vi "SamsGrapher.vi"() -> ()   [LabVIEW 2016]
uses:
  inventory type def.ctl
  Communication Global variables.vi
  <vilib>/addons/_JKI.lib/Serialization/JSON/JKI JSON Serialization.lvlib
panel:
  in  "Tab Control":enum32{"Controls", "Graph", "Help", "Fun"}(tab)
  in  "Load Config file":bool
  in  "Save Config file":bool
  in  "refresh list":bool
  in  "Device selection":i32(listbox)
  in  "Selected parameters":i32[](listbox)
  in  "Available parameters":i32[](listbox)
  in  "Config Button":bool
  out "Time range (Sec)":dbl format="%#.3g"
  in  "zoom out":bool
  in  "zoom in":bool
  out "Data rate (hz)":dbl(knob) scale=0.0..600.0
  in  "Enable graphing":bool=TRUE
  out "Waveform chart":waveform(dbl)[](graph)=[{"t0"=timestamp(742.987 s since 1904-01-01), "dt"=1.0, "Y"=[15300.0]}, {"t0"=timestamp(742.987 s since 1904-01-01), "dt"=1.0, "Y"=[15460.0]}, {"t0"=timestamp(742.987 s since 1904-01-01), "dt"=1.0, "Y"=[19658.0]}, {"t0"=timestamp(742.987 s since 1904-01-01), "dt"=1.0, "Y"=[18856.0]}]
  in  "stop":bool
  in  "Robor approved":u16(ring)
  in  "Robot Approved?":bool
  out "initialize error":errorcluster
  out "error out":errorcluster
  # "Parameter Selection"
  # "Xl Version 19.1.4"
  # "Click and drag \nselected parameters\nto change the order"
  # "Double click parameter name to add or remove it"
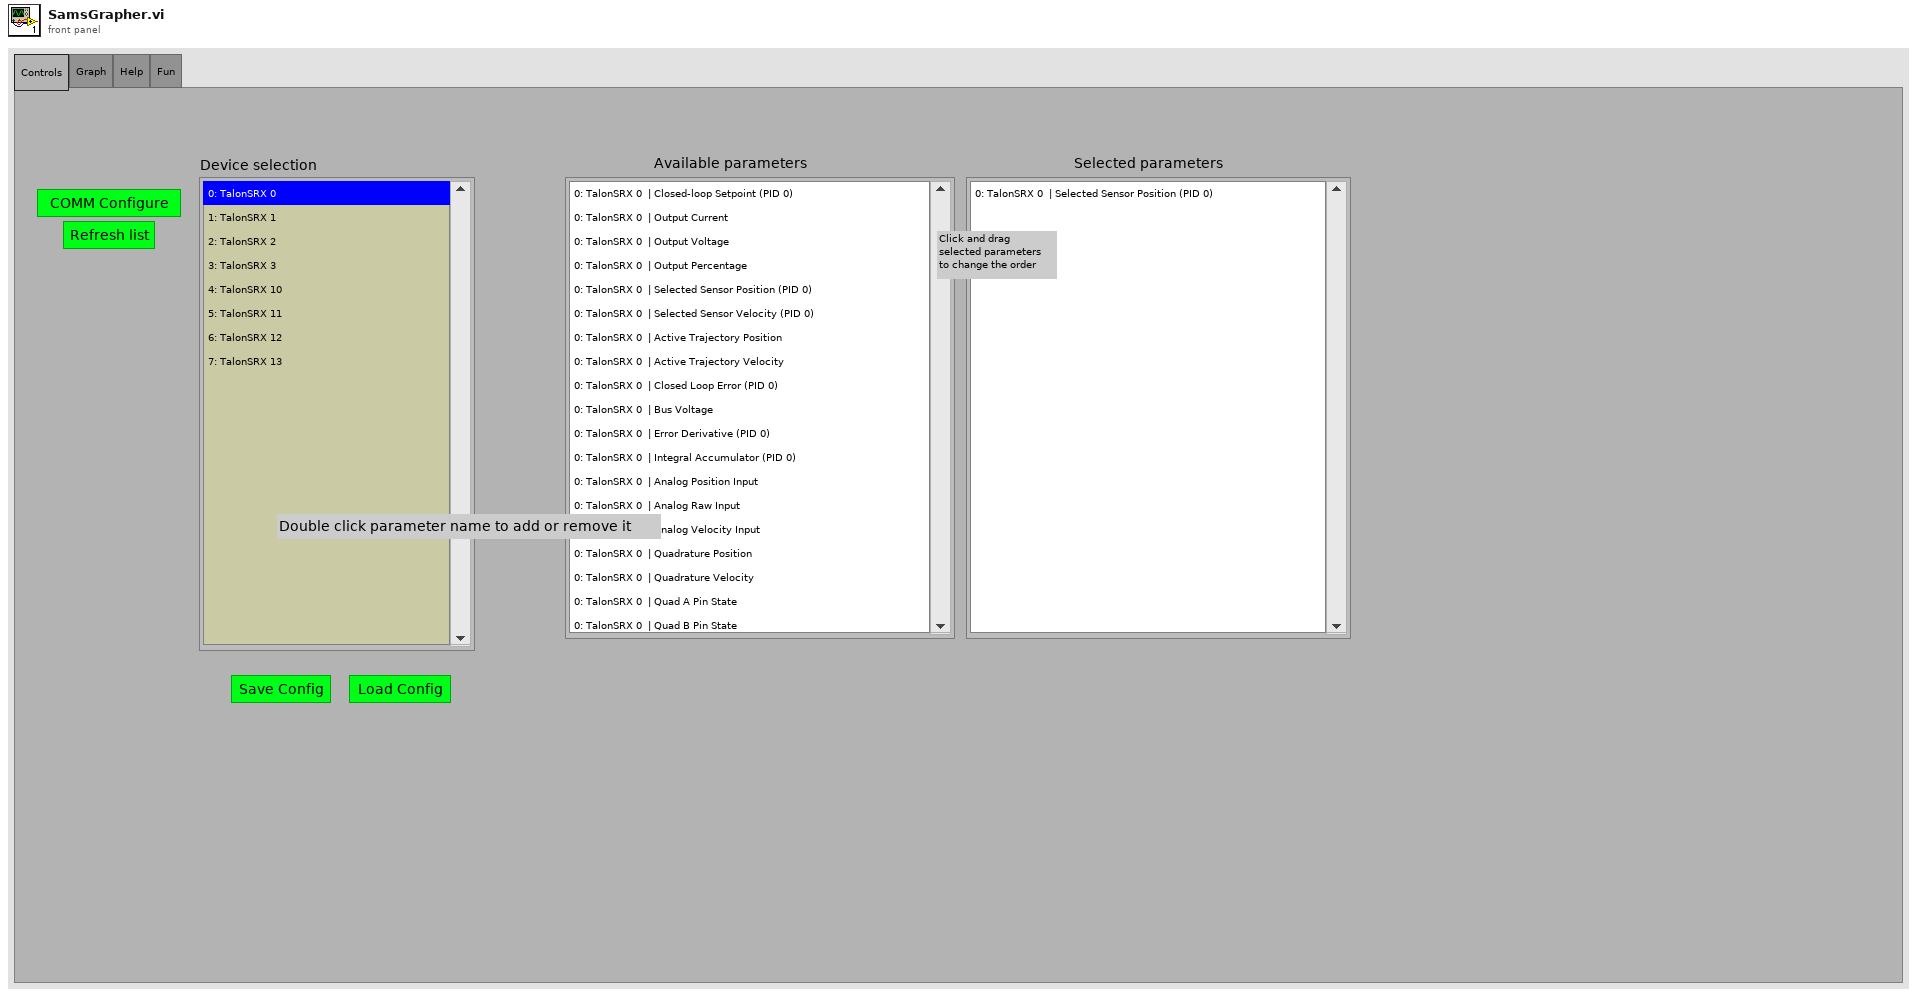
[diagram p1: front panel]
types:
  T1 = typedef "inventory type def.ctl" = cluster{"items":cluster{"id":u8, "type":string, "description":string}[], "measures":cluster{"deviceType":string, "deviceMeasures":cluster{"id":string, "description":string}[]}[], "type":string}
  T2 = enum8{"Enabled", "Disabled", "Disabled and Grayed Out"}
  T3 = cluster{"type":string, "timestamp":i64, "data":dbl[]}
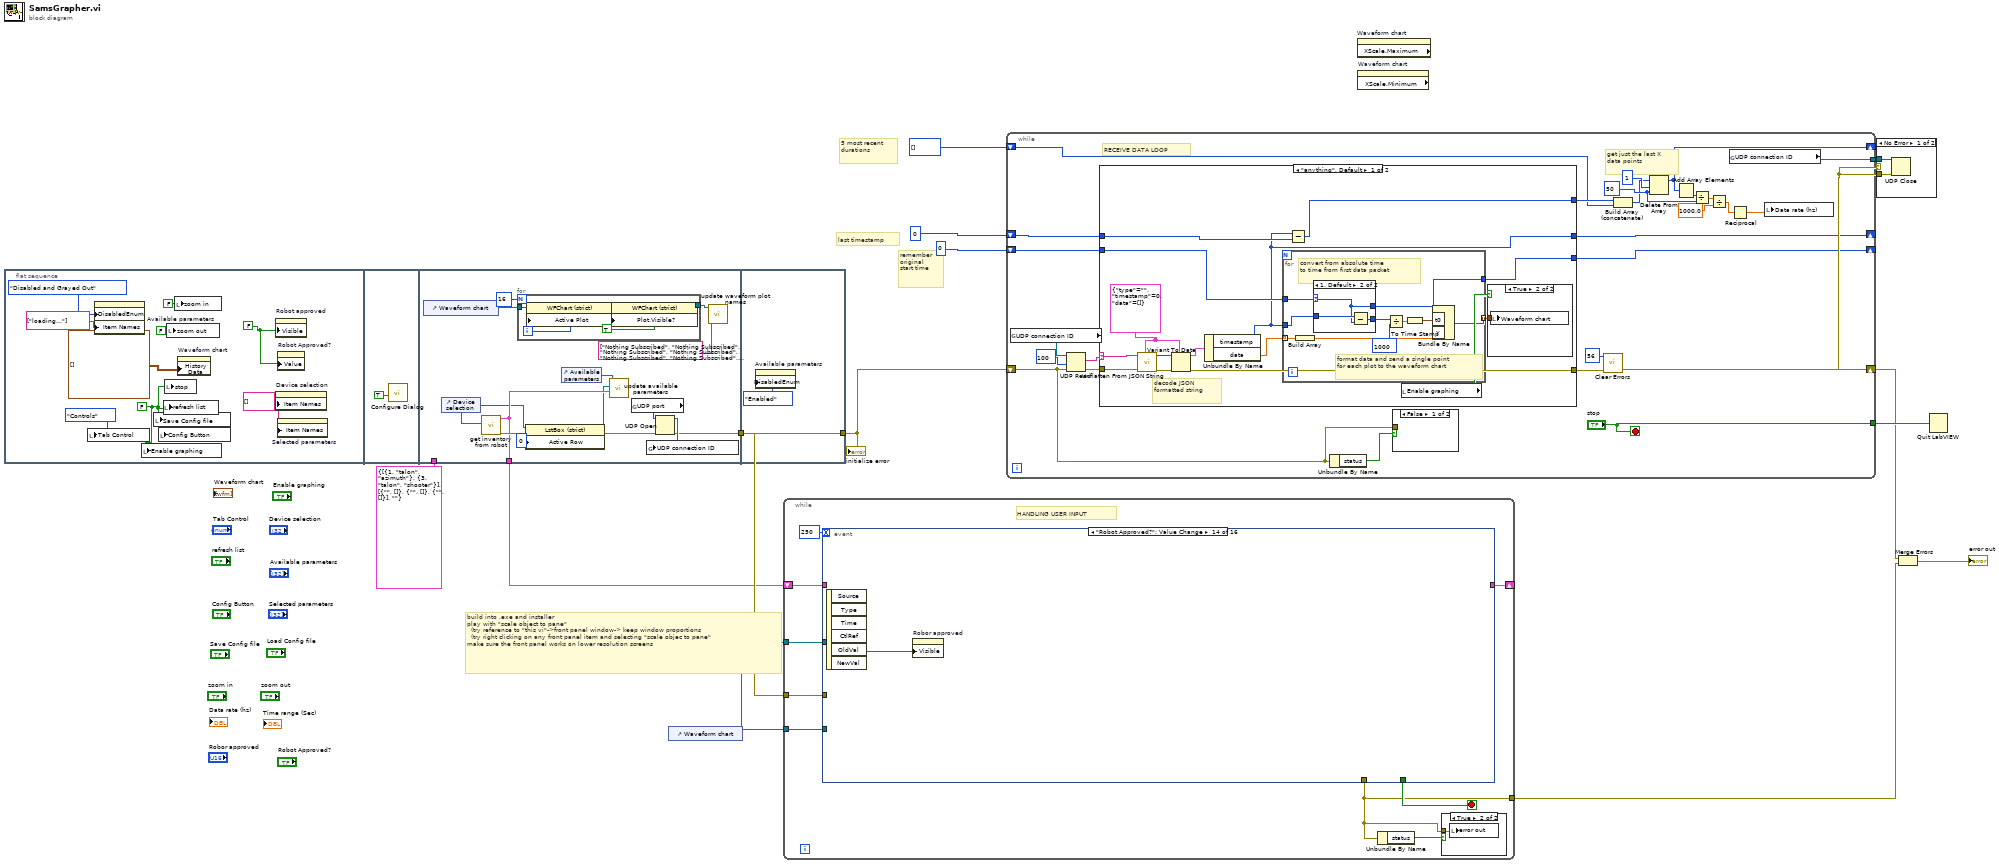
[diagram p0: block diagram]
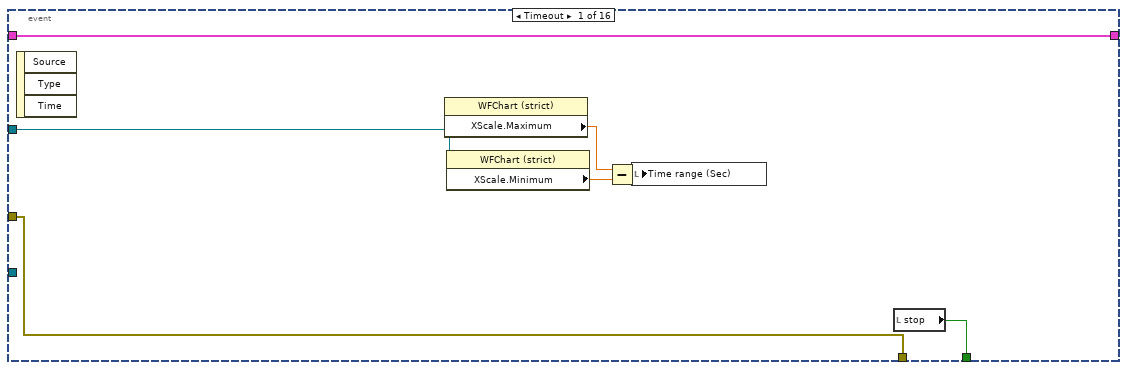
[diagram p4: hidden frame]
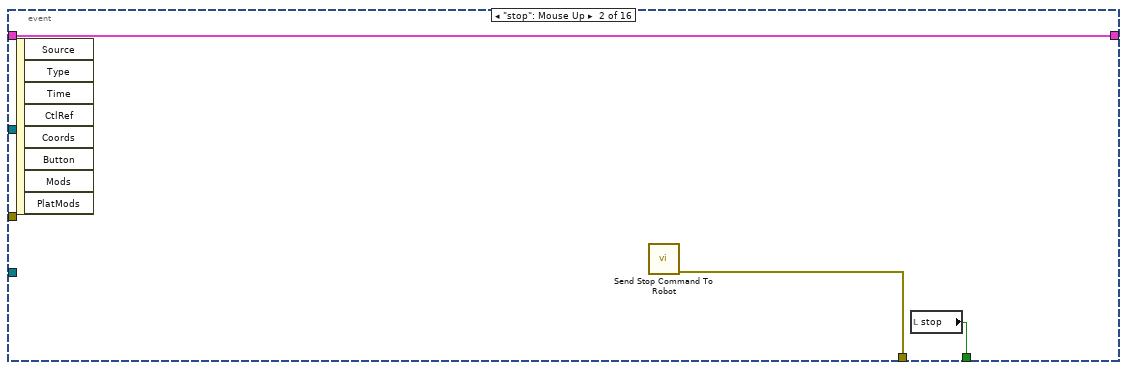
[diagram p5: hidden frame]
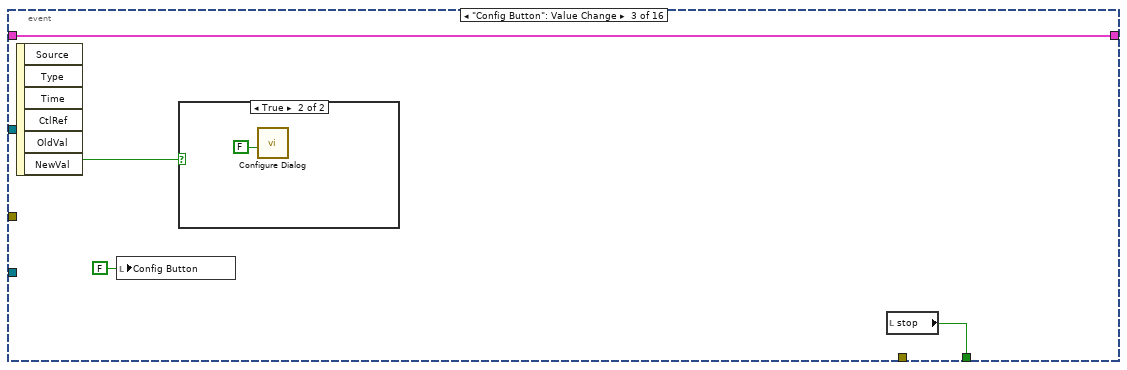
[diagram p6: hidden frame]
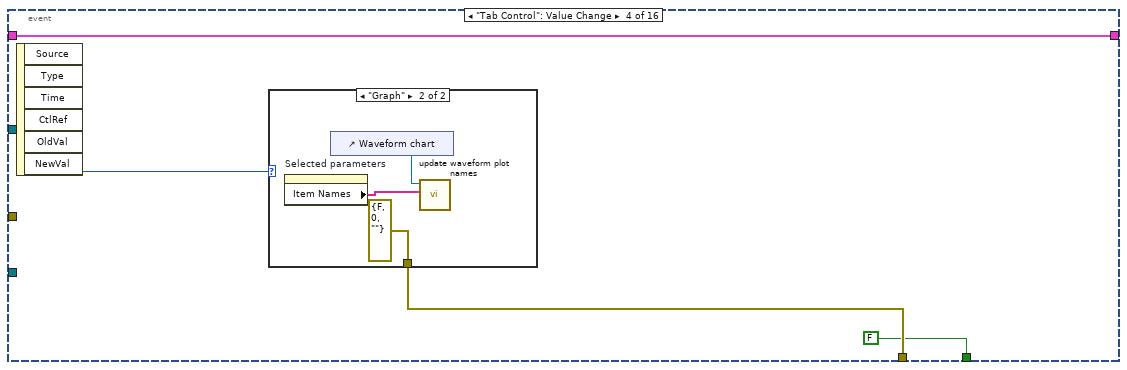
[diagram p8: hidden frame]
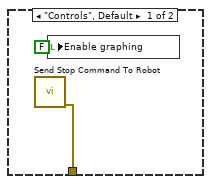
[diagram p9: hidden frame]
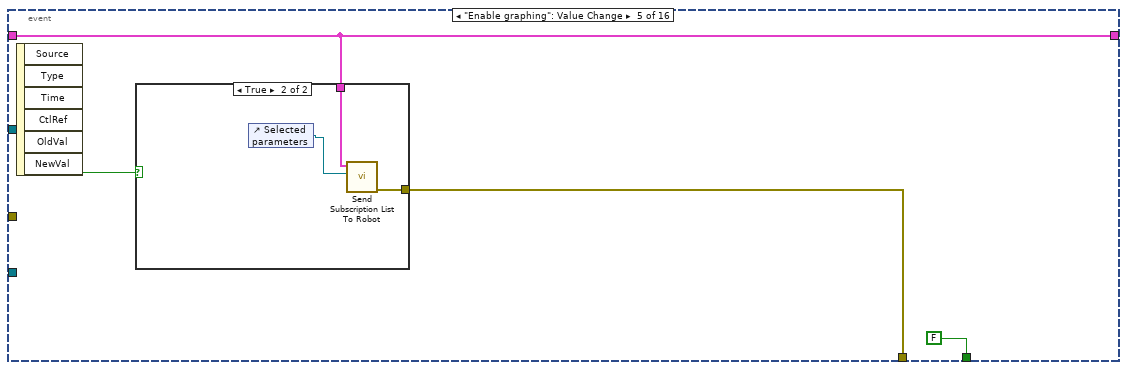
[diagram p10: hidden frame]
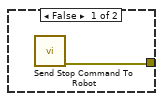
[diagram p11: hidden frame]
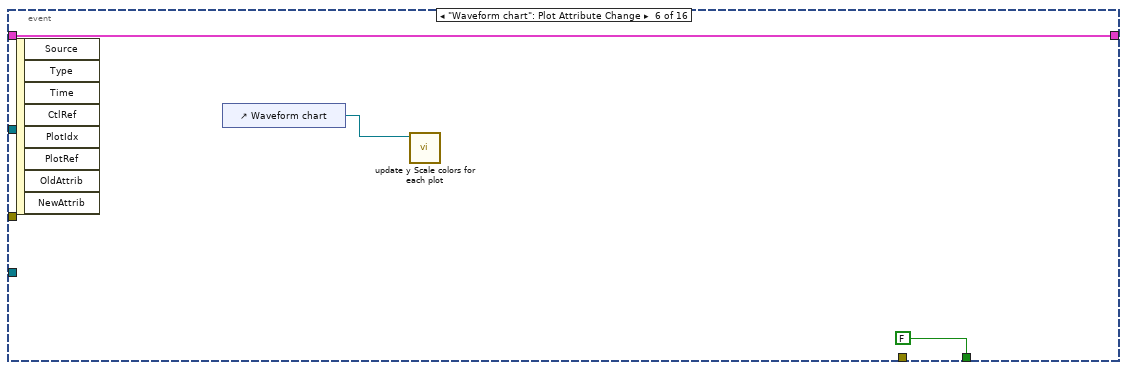
[diagram p12: hidden frame]
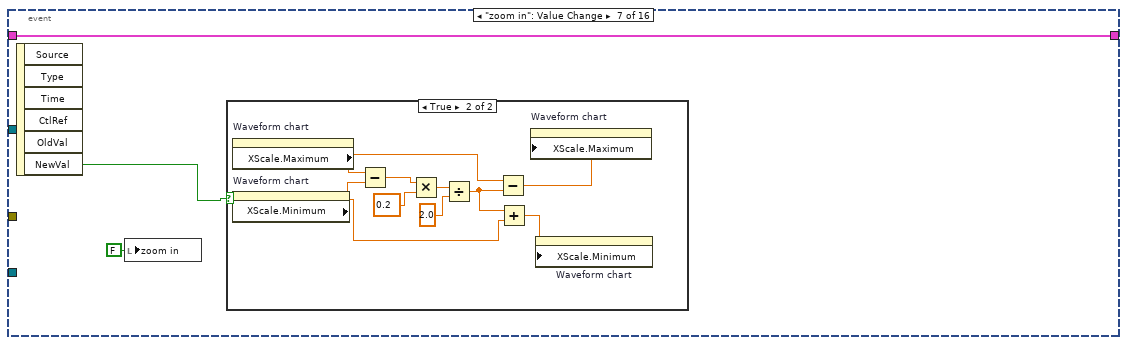
[diagram p13: hidden frame]
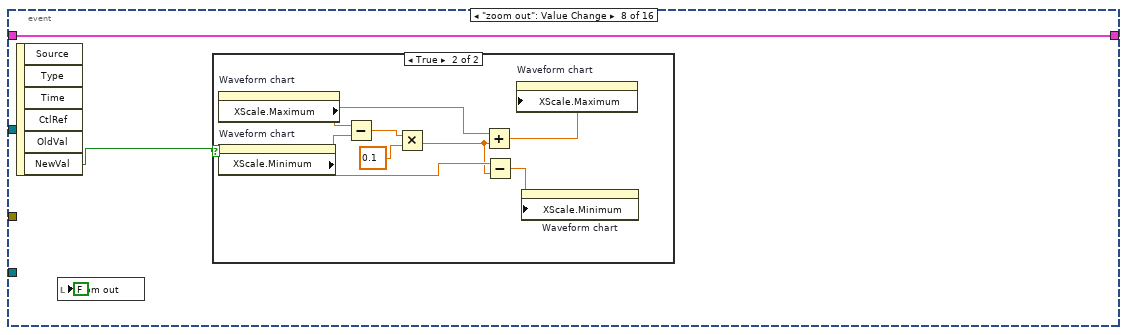
[diagram p15: hidden frame]
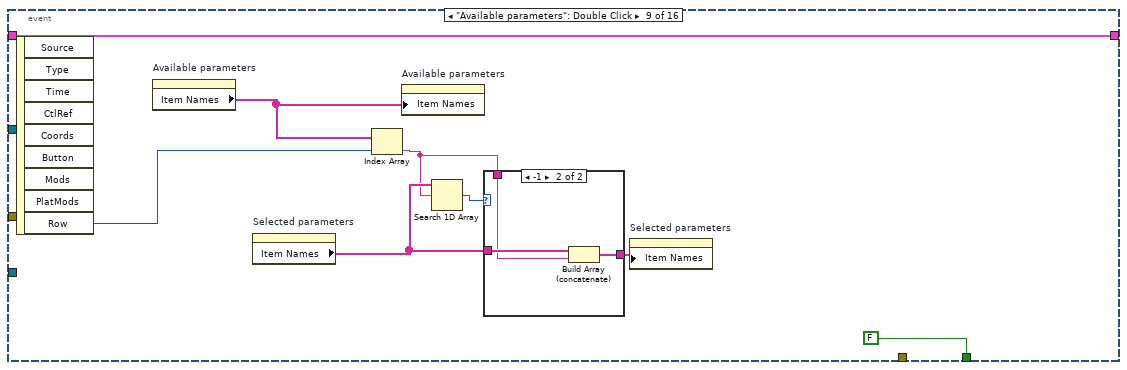
[diagram p17: hidden frame]
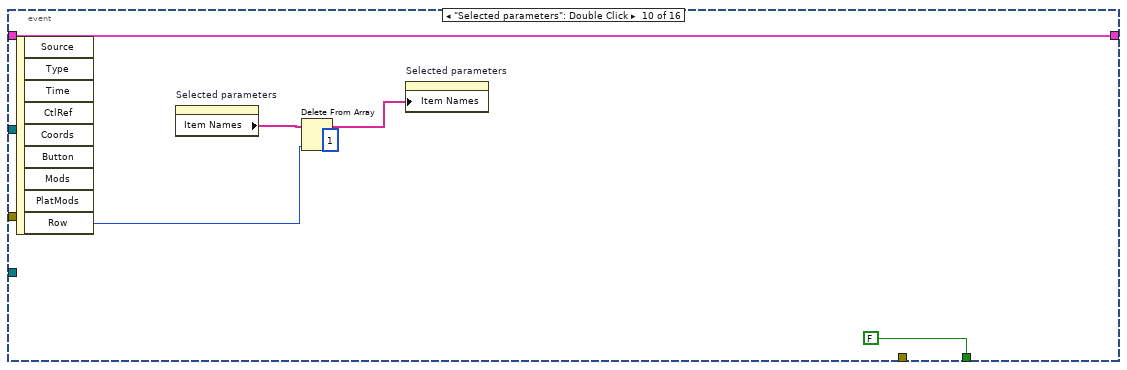
[diagram p19: hidden frame]
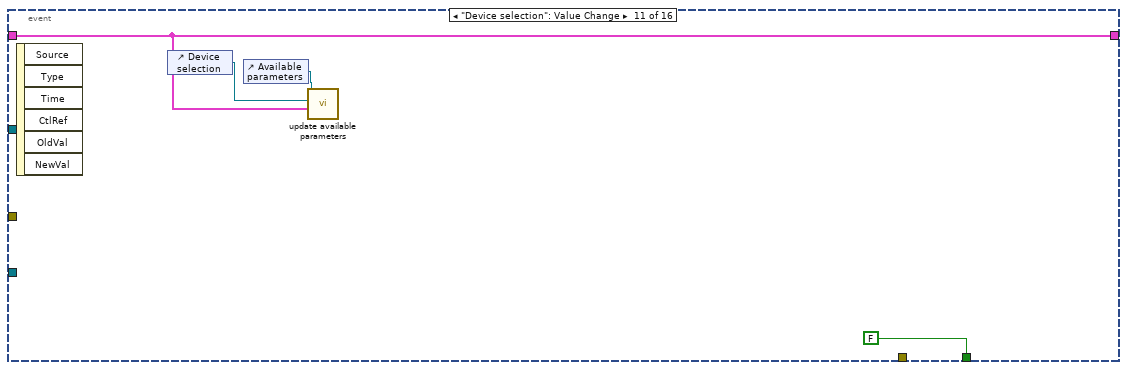
[diagram p20: hidden frame]
diagram:
  # "last timestamp"
  # "remember\noriginal\nstart time"
  # "5 most recent\ndurations"
  # "build into .exe and installer\nplay with \"scale object to pane\" \n  (try reference to \"this vi\"->front panel window-> keep window proportions\n  (try right clicking on any front panel item and selecting \"scale objec to pane\"\nmake sure the front panel works on lower resolution screens"
  n1 = flat-sequence {
    tunnel: [w26] -> w10
    tunnel: T1 {"items"=[{"id"=1, "type"="talon", "description"="azimuth"}, {"id"=3, "type"="talon", "description"="shooter"}], "measures"=[{"deviceType"="", "deviceMeasures"=[]}, {"deviceType"="", "deviceMeasures"=[]}, {"deviceType"="", "deviceMeasures"=[]}], "type"=""} -> [_]
    tunnel: [w35] -> w4
    tunnel: [w44] -> w11
    tunnel: w4 -> [w44]
    frame #0 {
      w14 = FALSE ("Visible")
      w15 = string[] [] ("Item Names")
      w21 = FALSE ("Send")
      n2 = local write "Tab Control"(enum32{"Controls", "Graph"}."Controls" ("Tab Control")) -> ()
      n3 = property on="Available parameters" class="LstBox (strict)"("DisabledEnum"=T2."Disabled and Grayed Out" ("Disabled"), "Item Names"=string[] ["loading..."]) -> ()  [unwired: 2 in, 2 out]
      n4 = local write "Enable graphing"(w21) -> ()
      n5 = local write "Save Config file"(w21) -> ()
      n6 = local write "Config Button"(w21) -> ()
      n7 = local write "refresh list"(w21) -> ()
      n8 = local write "stop"(w21) -> ()
      n9 = local write "zoom out"(FALSE ("zoom out")) -> ()
      n10 = local write "zoom in"(FALSE ("zoom in")) -> ()
      n11 = property on="Waveform chart" class="WFChart (strict)"("History Data"=waveform(dbl)[][] []) -> ()  [unwired: 2 in, 2 out]
      n12 = property on="Robot approved" class="Ring (strict)"("Visible"=w14) -> ()  [unwired: 2 in, 2 out]
      n13 = property on="Device selection" class="LstBox (strict)"("Item Names"=w15) -> ()  [unwired: 2 in, 2 out]
      n14 = property on="Robot Approved?" class="Bool (strict)"("Value"=w14) -> ()  [unwired: 2 in, 2 out]
      n15 = property on="Selected parameters" class="LstBox (strict)"("Item Names"=w15) -> ()  [unwired: 2 in, 2 out]
    }
    frame #1 {
      n16 = call "Configure Dialog.vi"("First time?"=TRUE) -> ()  [unwired: 10 in]
    }
    frame #2 {
      n17 = control-ref of="Waveform chart"() -> (w32:refnum<vi>)
      n18 = control-ref of="Device selection"() -> (w24:refnum<vi>)
      n19 = call "get inventory from robot.vi"("Device selection"=w24) -> ("error out"=w29:errorcluster, "Inventory"=w26:T1)  [unwired: 9 in]
      n20 = for {
        N: 16 -> [_]
        tunnel: w32 -> [w42]
        tunnel: [w38] -> w30
        i -> [w40]
        n21 = property class="WFChart (strict)"(reference=w42, "Active Plot"=w40) -> (reference out=w41:refnum<vi>)  [unwired: 1 in, 1 out]
        n22 = property class="WFChart (strict)"(reference=w41, "Plot.Visible?"=TRUE ("Plot.Visible")) -> (reference out=w38:refnum<vi>)  [unwired: 1 in, 1 out]
      }
      n23 = property class="LstBox (strict)"(reference=w24, error in=w29, "Active Row"=0 ("Active Row:Active Row Number")) -> (reference out=w25:refnum<vi>, error out=w28:errorcluster)
      n24 = control-ref of="Available parameters"() -> (w34:refnum<vi>)
      n25 = call "update available parameters.vi"("inventory"=w26, "Device selection"=w25, "Available parameters"=w34) -> ()  [unwired: 9 in]
      n26 = global read "Communication Global variables.vi" "UDP port"() -> (w36:u16)
      n27 = UDP Open(8:w28, 11:w36) -> (port=w37:refnum<k16>, 0:w35:errorcluster)  [unwired: 3 in, 1 out]
      n28 = global write "Communication Global variables.vi" "UDP connection ID"(w37) -> ()
      n29 = call "update waveform plot names.vi"("selected plot names"=string[] ["Nothing Subscribed", "Nothing Subscribed", "Nothing Subscribed", "Nothing Subscribed", "Nothing Subscribed", "Nothing Subscribed", "Nothing Subscribed", "Nothing Subscribed", "Nothing Subscribed", "Nothing Subscribed", "Nothing Subscribed", "Nothing Subscribed", "Nothing Subscribed", "Nothing Subscribed", "Nothing Subscribed", "Nothing Subscribed"], "WaveformChart in"=w30) -> ()  [unwired: 10 in]
    }
    frame #3 {
      n30 = property on="Available parameters" class="LstBox (strict)"("DisabledEnum"=T2."Enabled" ("Disabled")) -> ()  [unwired: 2 in, 2 out]
    }
  }
  n31 = control-ref of="Waveform chart"() -> (w1:refnum<vi>)
  n32 = while {
    tunnel: w11 -> [w52]
    shift-right: [w50] -> _
    shift-left: w10 -> [w51]
    tunnel: [w45] -> w8
    tunnel: w1 -> [w49]
    tunnel: w1 -> [w48]
    stop <- w47 stop-if-true
    # "HANDLING USER INPUT"
    n33 = event shown="[13] \"Robot Approved?\": Value Change" {
      selector: _ -> [_ _ _ _ _ _ _ _ _ _ _ _ _ _ _ _]
      dyn-events: _ -> [_ _ _ _ _ _ _ _ _ _ _ _ _ _ _ _]
      timeout: 250 -> [_ _ _ _ _ _ _ _ _ _ _ _ _ _ _ _]
      tunnel: [w61 w64 w67 FALSE ("stop") FALSE ("stop") FALSE ("stop") _ _ FALSE ("stop") FALSE ("stop") FALSE ("stop") FALSE ("stop") _ _ _ _] -> w47
      tunnel: w52 -> [w59 _ _ _ _ _ _ _ _ _ _ _ _ _ _ _]
      tunnel: w51 -> [w60 w63 w66 w70 w79 w89 w90 w102 w118 w125 w131 w134 w147 _ _ w183]
      tunnel: [w60 w63 w66 w70 w79 w89 w90 w102 w118 w125 w131 w135 w147 _ _ w183] -> w50
      tunnel: [w59 w62 _ w72 w81 _ _ _ _ _ _ _ _ _ _ _] -> w45
      tunnel: w49 -> [w55 _ _ _ _ _ _ _ _ _ _ _ _ _ _ _]
      tunnel: w48 -> [_ _ _ _ _ _ _ _ _ _ _ _ _ _ w153 _]
      event Timeout {
        n34 = event-data() -> ()  [unwired: 1 in, 3 out]
        n35 = property class="WFChart (strict)"(reference=w55) -> ("XScale.Maximum"=w57:dbl)  [unwired: 1 in, 2 out]
        n36 = property class="WFChart (strict)"(reference=w55) -> ("XScale.Minimum"=w56:dbl)  [unwired: 1 in, 2 out]
        n37 = Subtract(x=w57, y=w56) -> (x-y=w58:dbl)
        n38 = local write "Time range (Sec)"(w58) -> ()
        n39 = local read "stop"() -> (w61:bool)
      }
      event "stop": Mouse Up {
        n40 = event-data() -> ()  [unwired: 1 in, 8 out]
        n41 = call "Send Stop Command To Robot.vi"() -> ("error out"=w62:errorcluster)  [unwired: 11 in]
        n42 = local read "stop"() -> (w64:bool)
      }
      event "Config Button": Value Change {
        n43 = event-data() -> ("NewVal"=w65:bool)  [unwired: 1 in, 5 out]
        n44 = local write "Config Button"(FALSE ("Config Button")) -> ()
        n45 = case shown="True" w65 {
          frame False {
          }
          frame True {
            n46 = call "Configure Dialog.vi"("First time?"=FALSE) -> ()  [unwired: 10 in]
          }
        }
        n47 = local read "stop"() -> (w67:bool)
      }
      event "Tab Control": Value Change {
        n48 = event-data() -> ("NewVal"=w73:enum32{"Controls", "Graph", "Help", "Fun"})  [unwired: 1 in, 5 out]
        n49 = case shown="\"Graph\"" w73 {
          tunnel: [w75 errorcluster {"status"=FALSE, "code"=0, "source"=""} ("error out")] -> w72
          frame "Controls", Default {
            n50 = call "Send Stop Command To Robot.vi"() -> ("error out"=w75:errorcluster)  [unwired: 11 in]
            n51 = local write "Enable graphing"(FALSE ("Enable graphing")) -> ()
          }
          frame "Graph" {
            n52 = property on="Selected parameters" class="LstBox (strict)"() -> ("Item Names"=w77:string[])  [unwired: 2 in, 2 out]
            n53 = control-ref of="Waveform chart"() -> (w78:refnum<vi>)
            n54 = call "update waveform plot names.vi"("selected plot names"=w77, "WaveformChart in"=w78) -> ()  [unwired: 10 in]
          }
        }
      }
      event "Enable graphing": Value Change {
        n55 = event-data() -> ("NewVal"=w82:bool)  [unwired: 1 in, 5 out]
        n56 = case shown="True" w82 {
          tunnel: [w83 w86] -> w81
          tunnel: w79 -> [_ w84]
          frame False {
            n57 = call "Send Stop Command To Robot.vi"() -> ("error out"=w83:errorcluster)  [unwired: 11 in]
          }
          frame True {
            n58 = control-ref of="Selected parameters"() -> (w85:refnum<vi>)
            n59 = call "Send Subscription List To Robot.vi"("Selected parameters 2"=w85, "Inventory"=w84) -> ("error out"=w86:errorcluster)  [unwired: 9 in]
          }
        }
      }
      event "Waveform chart": Plot Attribute Change {
        n60 = event-data() -> ()  [unwired: 1 in, 8 out]
        n61 = control-ref of="Waveform chart"() -> (w88:refnum<vi>)
        n62 = call "update y Scale colors for each plot.vi"("WaveformChart in"=w88) -> ()  [unwired: 11 in]
      }
      event "zoom in": Value Change {
        n63 = event-data() -> ("NewVal"=w91:bool)  [unwired: 1 in, 5 out]
        n64 = local write "zoom in"(FALSE ("zoom in")) -> ()
        n65 = case shown="True" w91 {
          frame False {
          }
          frame True {
            n66 = property on="Waveform chart" class="WFChart (strict)"() -> ("XScale.Maximum"=w96:dbl)  [unwired: 2 in, 2 out]
            n67 = property on="Waveform chart" class="WFChart (strict)"() -> ("XScale.Minimum"=w95:dbl)  [unwired: 2 in, 2 out]
            n68 = Subtract(x=w96, y=w95) -> (x-y=w101:dbl)
            n69 = Multiply(x=w101, y=0.2) -> (x*y=w98:dbl)
            n70 = Divide(x=w98, y=2.0) -> (x/y=w93:dbl)
            n71 = Subtract(x=w96, y=w93) -> (x-y=w99:dbl)
            n72 = Add(x=w93, y=w95) -> (x+y=w94:dbl)
            n73 = property on="Waveform chart" class="WFChart (strict)"("XScale.Maximum"=w99) -> ()  [unwired: 2 in, 2 out]
            n74 = property on="Waveform chart" class="WFChart (strict)"("XScale.Minimum"=w94) -> ()  [unwired: 2 in, 2 out]
          }
        }
      }
      event "zoom out": Value Change {
        n75 = event-data() -> ("NewVal"=w103:bool)  [unwired: 1 in, 5 out]
        n76 = local write "zoom out"(FALSE ("zoom out")) -> ()
        n77 = case shown="True" w103 {
          frame False {
          }
          frame True {
            n78 = property on="Waveform chart" class="WFChart (strict)"() -> ("XScale.Maximum"=w108:dbl)  [unwired: 2 in, 2 out]
            n79 = property on="Waveform chart" class="WFChart (strict)"() -> ("XScale.Minimum"=w106:dbl)  [unwired: 2 in, 2 out]
            n80 = Subtract(x=w108, y=w106) -> (x-y=w111:dbl)
            n81 = Multiply(x=w111, y=0.1) -> (x*y=w105:dbl)
            n82 = Add(x=w108, y=w105) -> (x+y=w109:dbl)
            n83 = Subtract(x=w106, y=w105) -> (x-y=w107:dbl)
            n84 = property on="Waveform chart" class="WFChart (strict)"("XScale.Maximum"=w109) -> ()  [unwired: 2 in, 2 out]
            n85 = property on="Waveform chart" class="WFChart (strict)"("XScale.Minimum"=w107) -> ()  [unwired: 2 in, 2 out]
          }
        }
      }
      event "Available parameters": Double Click {
        n86 = event-data() -> ("Row"=w112:i32)  [unwired: 1 in, 8 out]
        n87 = property on="Available parameters" class="LstBox (strict)"() -> ("Item Names"=w113:string[])  [unwired: 2 in, 2 out]
        n88 = property on="Selected parameters" class="LstBox (strict)"() -> ("Item Names"=w116:string[])  [unwired: 2 in, 2 out]
        n89 = Index Array(array=w113, index=w112) -> (element=w114:string)
        n90 = property on="Available parameters" class="LstBox (strict)"("Item Names"=w113) -> ()  [unwired: 2 in, 2 out]
        n91 = Search 1D Array(1D array=w116, element=w114) -> (index of element=w115:i32)  [unwired: 1 in]
        n92 = case shown="-1" w115 {
          tunnel: [w120 w123] -> w119
          tunnel: w116 -> [w120 w122]
          tunnel: w114 -> [_ w121]
          frame 0, Default {
          }
          frame -1 {
            n93 = Build Array (concatenate)(w122, w121) -> (w123:string[])
          }
        }
        n94 = property on="Selected parameters" class="LstBox (strict)"("Item Names"=w119) -> ()  [unwired: 2 in, 2 out]
      }
      event "Selected parameters": Double Click {
        n95 = event-data() -> ("Row"=w127:i32)  [unwired: 1 in, 8 out]
        n96 = property on="Selected parameters" class="LstBox (strict)"() -> ("Item Names"=w129:string[])  [unwired: 2 in, 2 out]
        n97 = Delete From Array(array=w129, length=1, index=w127) -> (array with subset deleted=w126:string[])  [unwired: 1 out]
        n98 = property on="Selected parameters" class="LstBox (strict)"("Item Names"=w126) -> ()  [unwired: 2 in, 2 out]
      }
      event "Device selection": Value Change {
        n99 = event-data() -> ()  [unwired: 1 in, 6 out]
        n100 = control-ref of="Device selection"() -> (w130:refnum<vi>)
        n101 = control-ref of="Available parameters"() -> (w133:refnum<vi>)
        n102 = call "update available parameters.vi"("inventory"=w131, "Device selection"=w130, "Available parameters"=w133) -> ()  [unwired: 9 in]
      }
      event "refresh list": Value Change {
        n103 = event-data() -> ("NewVal"=w138:bool)  [unwired: 1 in, 5 out]
        n104 = case shown="True" w138 {
          tunnel: [w139 w140] -> w135
          tunnel: w134 -> [w139 _]
          frame False {
          }
          frame True {
            n105 = flat-sequence {
              tunnel: [w143] -> w140
              frame #0 {
                n106 = property on="Available parameters" class="LstBox (strict)"("DisabledEnum"=T2."Disabled and Grayed Out" ("Disabled"), "Item Names"=string[] ["Loading..."]) -> ()  [unwired: 2 in, 2 out]
              }
              frame #1 {
                n107 = control-ref of="Device selection"() -> (w144:refnum<vi>)
                n108 = call "get inventory from robot.vi"("Device selection"=w144) -> ("Inventory"=w143:T1)  [unwired: 9 in, 1 out]
                n109 = control-ref of="Available parameters"() -> (w145:refnum<vi>)
                n110 = call "update available parameters.vi"("inventory"=w143, "Device selection"=w144, "Available parameters"=w145) -> ()  [unwired: 9 in]
              }
              frame #2 {
                n111 = property on="Available parameters" class="LstBox (strict)"("DisabledEnum"=T2."Enabled" ("Disabled")) -> ()  [unwired: 2 in, 2 out]
              }
            }
          }
        }
        n112 = local write "refresh list"(FALSE ("refresh list")) -> ()
      }
      event "Save Config file": Value Change {
        n113 = event-data() -> ("NewVal"=w149:bool)  [unwired: 1 in, 5 out]
        n114 = local write "Save Config file"(FALSE ("Save Config")) -> ()
        n115 = case shown="True" w149 {
          frame False {
          }
          frame True {
            n116 = control-ref of="Waveform chart"() -> (w150:refnum<vi>)
            n117 = property on="Selected parameters" class="LstBox (strict)"() -> ("Item Names"=w151:string[])  [unwired: 2 in, 2 out]
            n118 = call "save configuration.vi"("Waveform chart"=w150, "selected parameters"=w151) -> ()  [unwired: 10 in]
          }
        }
      }
      event "Robot Approved?": Value Change {
        n119 = event-data() -> ("NewVal"=w152:bool)  [unwired: 1 in, 5 out]
        n120 = property on="Robor approved" class="Ring (strict)"("Visible"=w152) -> ()  [unwired: 2 in, 2 out]
      }
      event "Waveform chart": Mouse Wheel {
        n121 = event-data() -> ("Delta"=w154:i32)  [unwired: 1 in, 9 out]
        n122 = Greater?(x=w154, y=0.0) -> (0:w155:bool)
        n123 = for {
          N: 5 -> [_]
          tunnel: w153 -> [w169]
          tunnel: w155 -> [w158]
          i -> [w170]
          n124 = property class="WFChart (strict)"(reference=w169, "ActYScl"=w170) -> (reference out=w159:refnum<vi>)  [unwired: 1 in, 1 out]
          n125 = property on="Property Node" class="WFChart (strict)"(reference=w159) -> ("YScale.Minimum"=w163:dbl)  [unwired: 1 in, 2 out]
          n126 = property on="Property Node" class="WFChart (strict)"(reference=w159) -> ("YScale.Maximum"=w164:dbl)  [unwired: 1 in, 2 out]
          n127 = Subtract(x=w164, y=w163) -> (x-y=w168:dbl)
          n128 = Multiply(x=w168, y=0.2) -> (x*y=w166:dbl)
          n129 = Divide(x=w166, y=2.0) -> (x/y=w162:dbl)
          n130 = case shown="False" w158 {
            tunnel: w164 -> [w175 w180]
            tunnel: w163 -> [w172 w179]
            tunnel: w162 -> [w171 w178]
            tunnel: [w173 w177] -> w161
            tunnel: [w174 w176] -> w160
            frame False {
              n131 = Add(x=w175, y=w171) -> (x+y=w174:dbl)
              n132 = Subtract(x=w172, y=w171) -> (x-y=w173:dbl)
            }
            frame True {
              n133 = Add(x=w178, y=w179) -> (x+y=w177:dbl)
              n134 = Subtract(x=w180, y=w178) -> (x-y=w176:dbl)
            }
          }
          n135 = property on="Property Node" class="WFChart (strict)"(reference=w159, "YScale.Maximum"=w160) -> ()  [unwired: 1 in, 2 out]
          n136 = property on="Property Node" class="WFChart (strict)"(reference=w159, "YScale.Minimum"=w161) -> ()  [unwired: 1 in, 2 out]
        }
      }
      event "Load Config file": Value Change {
        n137 = event-data() -> ("NewVal"=w181:bool)  [unwired: 1 in, 5 out]
        n138 = local write "Load Config file"(FALSE ("Load Config file")) -> ()
        n139 = case shown="True" w181 {
          frame False {
          }
          frame True {
            n140 = control-ref of="Waveform chart"() -> (w186:refnum<vi>)
            n141 = call "load configuration file.vi"("Waveform chart"=w186) -> ("selected parameters"=w184:string[], "Waveform chart OUT"=w185:refnum<vi>)  [unwired: 9 in]
            n142 = property on="Selected parameters" class="LstBox (strict)"("Item Names"=w184) -> ()  [unwired: 2 in, 2 out]
            n143 = call "update y Scale colors for each plot.vi"("WaveformChart in"=w185) -> ()  [unwired: 11 in]
          }
        }
      }
    }
    n144 = Unbundle By Name(w45) -> ("status"=w46:bool)
    n145 = case shown="True" w46 {
      tunnel: w45 -> [_ w54]
      frame False {
      }
      frame True {
        n146 = local write "error out"(w54) -> ()
      }
    }
  }
  n147 = while {
    shift-right: [w212] -> w2
    shift-left: w11 -> [w188]
    tunnel: [w205] -> w12
    shift-right: [w203] -> _
    shift-left: i64 0 ("timestamp") -> [w204]
    shift-right: [w190] -> _
    shift-left: i64[] [] -> [w191]
    shift-right: [w201] -> _
    shift-left: i64 0 ("timestamp") -> [w202]
    tunnel: ["stop"] -> w3
    stop <- "stop" stop-if-true
    w196 = 50 ("index")
    # "get just the last X\ndata points"
    # "RECEIVE DATA LOOP"
    n148 = global read "Communication Global variables.vi" "UDP connection ID"() -> (w206:refnum<k16>)
    n149 = UDP Read(connection ID=w206, timeout ms (25000)=100, 8:w188) -> (data out=w209:string, error out=w210:errorcluster)  [unwired: 1 in, 3 out]
    n150 = case shown="\"anything\", Default" w209 {
      selector: w209 -> [w227 _]
      tunnel: w210 -> [w228 w248]
      tunnel: [w224 w248] -> w207
      tunnel: w204 -> [w218 w247]
      tunnel: [w217 w247] -> w203
      tunnel: w202 -> [w216 w246]
      tunnel: [w215 w246] -> w201
      tunnel: [w214 i64 1000] -> w192
      frame "anything", Default {
        w221 = T3 {"type"="", "timestamp"=0, "data"=[]}
        # "decode JSON\nformatted string"
        n151 = call <vilib>:"Unflatten From JSON String.vi"("Type and Defaults"=w221, "error in (no error)"=w228, "JSON String"=w227) -> ("error out"=w226:errorcluster, "Variant"=w225:variant)  [unwired: 7 in]
        n152 = Variant To Data(error in=w226, type=w221, Variant=w225) -> (data=w223:T3, error out=w224:errorcluster)
        n153 = Unbundle By Name(w223) -> ("timestamp"=w215:i64, "data"=w222:dbl[])
        n154 = for {
          tunnel: w215 -> [w235]
          tunnel: [w238] -> w219 mode=indexing
          tunnel: w222 -> [w237] mode=indexing
          tunnel: w218 -> [w234]
          tunnel: [w233] -> w217
          # "convert from absolute time\nto time from first data packet"
          # "format data and send a single point\nfor each plot to the waveform chart"
          n155 = Build Array(w237) -> (w239:dbl[])
          n156 = case shown="1, Default" w234 {
            selector: w234 -> [w241 w242]
            tunnel: [w241 w244] -> w230
            tunnel: w235 -> [w240 w243]
            tunnel: [w240 w242] -> w233
            frame 0 {
            }
            frame 1, Default {
              n157 = Subtract(x=w243, y=w242) -> (x-y=w244:i64)
            }
          }
          n158 = Divide(x=w230, y=i64 1000) -> (x/y=w232:dbl)
          n159 = To Time Stamp(1:w232) -> (0:w236:timestamp)
          n160 = Bundle By Name("t0"=w236, "Y"=w239) -> (w238:waveform(dbl))  [unwired: 1 in]
        }
        n161 = Subtract(x=w215, y=w216) -> (x-y=w214:i64)
        n162 = local read "Enable graphing"() -> (w220:bool)
        n163 = case shown="True" w220 {
          tunnel: w219 -> [_ w229]
          frame False {
          }
          frame True {
            n164 = local write "Waveform chart"(w229) -> ()
          }
        }
      }
      frame "" {
        # "if no data, put in\nsomething big"
      }
    }
    n165 = Unbundle By Name(w188) -> ("status"=w189:bool)
    n166 = case shown="False" w189 {
      tunnel: w188 -> [_ w213]
      frame False {
      }
      frame True {
        n167 = local write "error out"(w213) -> ()
      }
    }
    n168 = call <vilib>:"Clear Errors.vi"("error in (no error)"=w207, "specific error code to clear (0: all)"=56) -> ("error out"=w212:errorcluster)  [unwired: 4 in, 1 out]
    n169 = Build Array (concatenate)(w192, w191) -> (w193:i64[])
    n170 = Delete From Array(array=w193, length=1, index=w196) -> (array with subset deleted=w190:i64[])  [unwired: 1 out]
    n171 = Add Array Elements(numeric array=w190) -> (sum=w195:i64)
    n172 = Divide(x=w195, y=w196) -> (x/y=w197:dbl)
    n173 = Divide(x=w197, y=1000.0) -> (x/y=w199:dbl)
    n174 = global read "Communication Global variables.vi" "UDP connection ID"() -> (w205:refnum<k16>)
    n175 = Reciprocal(x=w199) -> (1/x=w200:dbl)
    n176 = local write "Data rate (hz)"(w200) -> ()
  }
  n177 = property on="Waveform chart" class="WFChart (strict)" props=["XScale", "Maximum"]() -> ()  [unwired: 2 in, 3 out]
  n178 = property on="Waveform chart" class="WFChart (strict)" props=["XScale", "Minimum"]() -> ()  [unwired: 2 in, 3 out]
  n179 = case shown="No Error" w2 {
    tunnel: w12 -> [w250 _]
    tunnel: w2 -> [w249 _]
    frame No Error {
      n180 = UDP Close(connection ID=w250, 8:w249) -> ()  [unwired: 2 out]
    }
    frame Error {
    }
  }
  n181 = Merge Errors(w2, w8) -> (→"error out":errorcluster)
  n182 = Quit LabVIEW(quit? (T)=w3) -> ()
  "initialize error" <- w11
